vi "求根公式.vi"(7 "A":dbl, 10 "C":dbl, 11 "B":dbl) -> (2 "X2":dbl, 3 "X1":dbl)   [LabVIEW 2018]
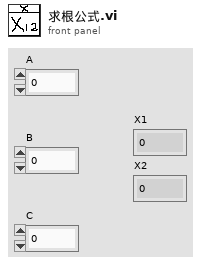
[diagram p1: front panel]
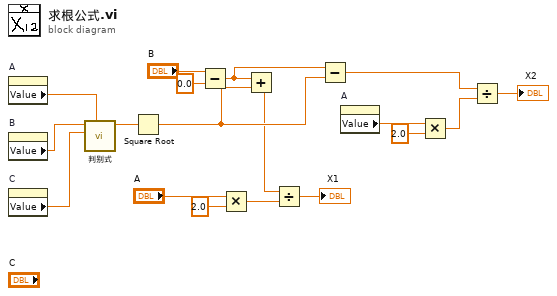
[diagram p0: block diagram]
diagram:
  n1 = property on="A" class="DigNum (严格)"() -> ("Value"=w16:dbl)  [unwired: 2 in, 2 out]
  n2 = property on="B" class="DigNum (严格)"() -> ("Value"=w15:dbl)  [unwired: 2 in, 2 out]
  n3 = property on="C" class="DigNum (严格)"() -> ("Value"=w14:dbl)  [unwired: 2 in, 2 out]
  n4 = call "判别式.vi"("A"=w16, "C"=w14, "B"=w15) -> ("判别式"=w13:dbl)  [unwired: 8 in]
  n5 = Square Root(x=w13) -> (sqrt(x)=w11:dbl)
  n6 = Subtract(x="B", y=0.0) -> (x-y=w12:dbl)
  n7 = Multiply(x="A", y=2.0) -> (x*y=w8:dbl)
  n8 = Add(x=w12, y=w11) -> (x+y=w7:dbl)
  n9 = Divide(x=w7, y=w8) -> (x/y=→"X1":dbl)
  n10 = Subtract(x=w12, y=w11) -> (x-y=w3:dbl)
  n11 = property on="A" class="DigNum (严格)"() -> ("Value"=w5:dbl)  [unwired: 2 in, 2 out]
  n12 = Multiply(x=w5, y=2.0) -> (x*y=w2:dbl)
  n13 = Divide(x=w3, y=w2) -> (x/y=→"X2":dbl)
